vi "live view D01.vi"() -> ()   [LabVIEW 2019, in "D01.lvlib"]
uses:
  D01.lvlib
  <vilib>/userDefined/High Color/IMAQdx.ctl
  <vilib>/vision/Image Controls.llb/IMAQ Image.ctl
  <vilib>/measure/mamon.llb/Trigger Detection for 1 Channel.vi
  <vilib>/measure/NI_MAPro.lvlib
  Calibration Lib.lvlib
  database.lvlib
  <vilib>/vision/driver/NI_Vision_Acquisition_Software.lvlib
panel:
  in  "Verify Calibration1 D01":bool caption="capture grab"
  in  "snapshot":bool
  out "error prj26":errorcluster
  in  "Path":path
  in  "Verify Calibration D01":bool caption="capture grab"
  in  "Close":bool
  in  "Method 2 save D01":bool caption="capture grab"
  in  "Method 1 Save D01":bool caption="Saving txt"
  out "Average Result":string="Average Result"
  out ">18  A":dbl(slide)=1.0 caption=">18 mm" scale=0.0..100.0
  out "16-18  A":dbl(slide)=1.0 caption="16-18 mm" scale=0.0..100.0
  out "14-16  A":dbl(slide)=1.0 caption="14-16 mm" scale=0.0..100.0
  out "12.5-14 A":dbl(slide)=1.0 caption="12.5-14 mm" scale=0.0..100.0
  out "10-12.5  A":dbl(slide)=1.0 caption="10-12.5 mm" scale=0.0..100.0 scale format="%#_4f"
  out "8-10  A":dbl(slide)=1.0 caption="8-10 mm" scale=0.0..100.0
  out "6.3-8  A":dbl(slide)=1.0 caption="6.3-8 mm" scale=0.0..100.0
  out "<6.3  A":dbl(slide)=1.0 caption="<6.3 mm" scale=0.0..100.0
  out "Live Result":string="Live Result"
  out ">18  L":dbl(slide)=1.0 caption=">18 mm" scale=0.0..100.0
  out "Live View":T1(plugin-control) caption="Disc 26"
  out "16-18  L":dbl(slide)=1.0 caption="16-18 mm" scale=0.0..100.0
  out "14-16  L":dbl(slide)=1.0 caption="14-16 mm" scale=0.0..100.0
  out "12.5-14 L":dbl(slide)=1.0 caption="12.5-14 mm" scale=0.0..100.0
  out "10-12.5  L":dbl(slide)=1.0 caption="10-12.5 mm" scale=0.0..100.0 scale format="%#_4f"
  out "8-10  L":dbl(slide)=1.0 caption="8-10 mm" scale=0.0..100.0
  out "6.3-8  L":dbl(slide)=1.0 caption="6.3-8 mm" scale=0.0..100.0
  out "<6.3  L":dbl(slide)=1.0 caption="<6.3 mm" scale=0.0..100.0
  out "disc name":string="Live Info Disc 01"
  out "dsgs":string="DSGS"
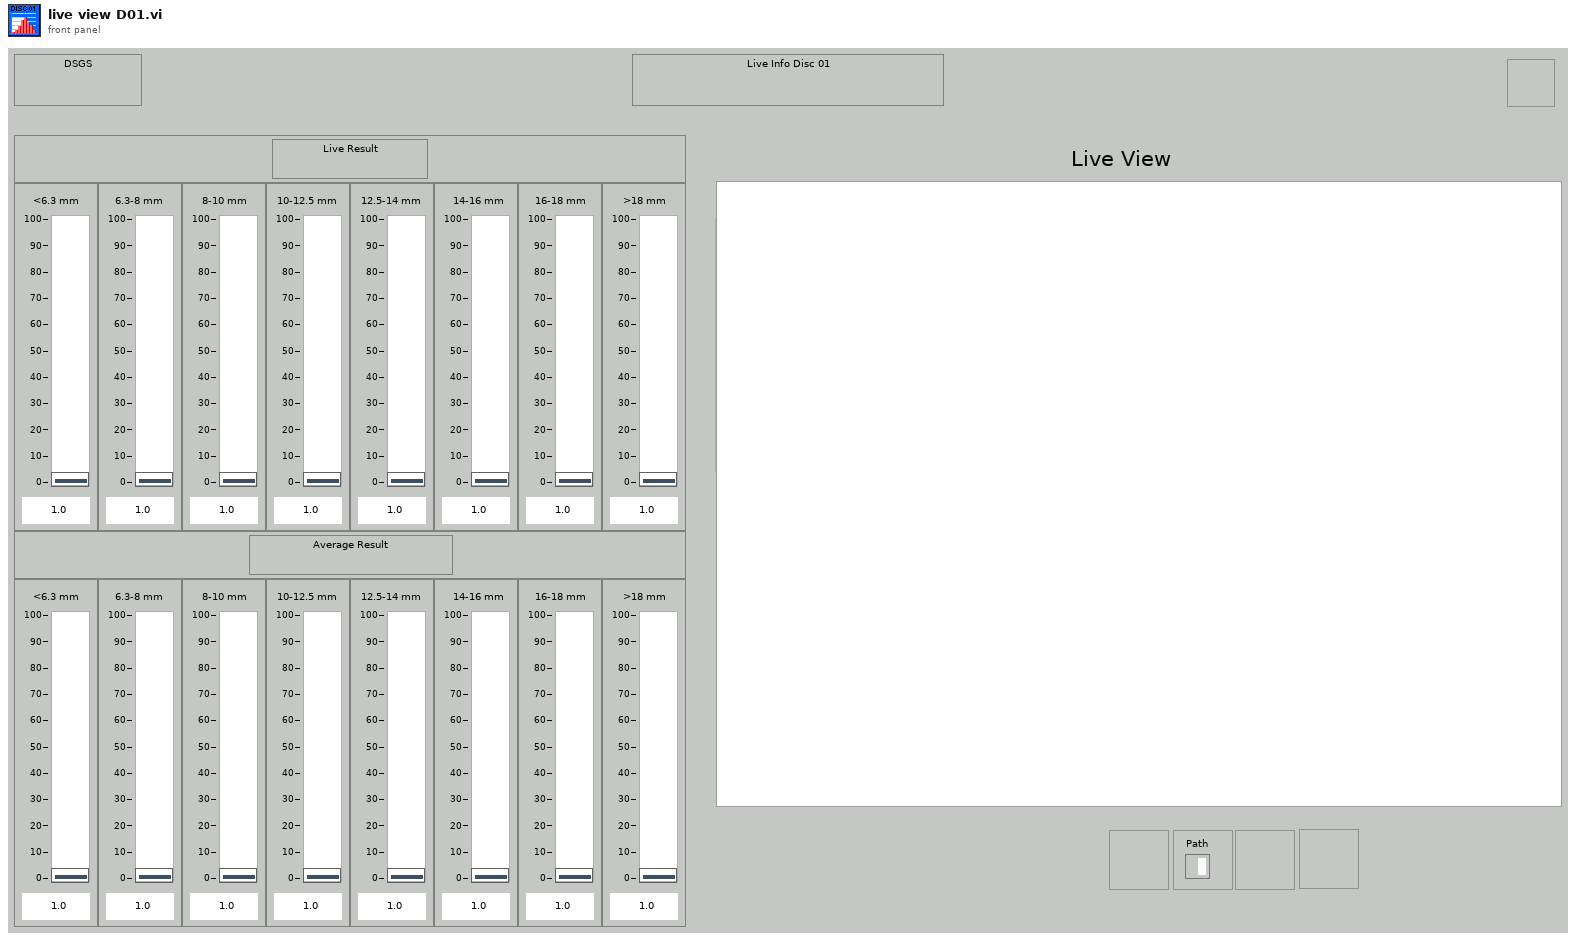
[diagram p1: front panel]
types:
  T1 = typedef "IMAQ Image.ctl" = refnum<image>
  T2 = typedef "IMAQdx.ctl" = refnum<k21>
  T3 = enum8{"Enabled", "Disabled", "Disabled and Grayed Out"}
  T4 = cluster{"date/time string":string, "date/time string":string, "date/time string":string, string, "spreadsheet string":string, string}
  T5 = cluster{"date/time string":string, "date/time string":string, string, "Value":dbl, "Value":dbl, "Value":dbl, "Value":dbl, "Value":dbl, "Value":dbl, "Value":dbl, "Value":dbl}
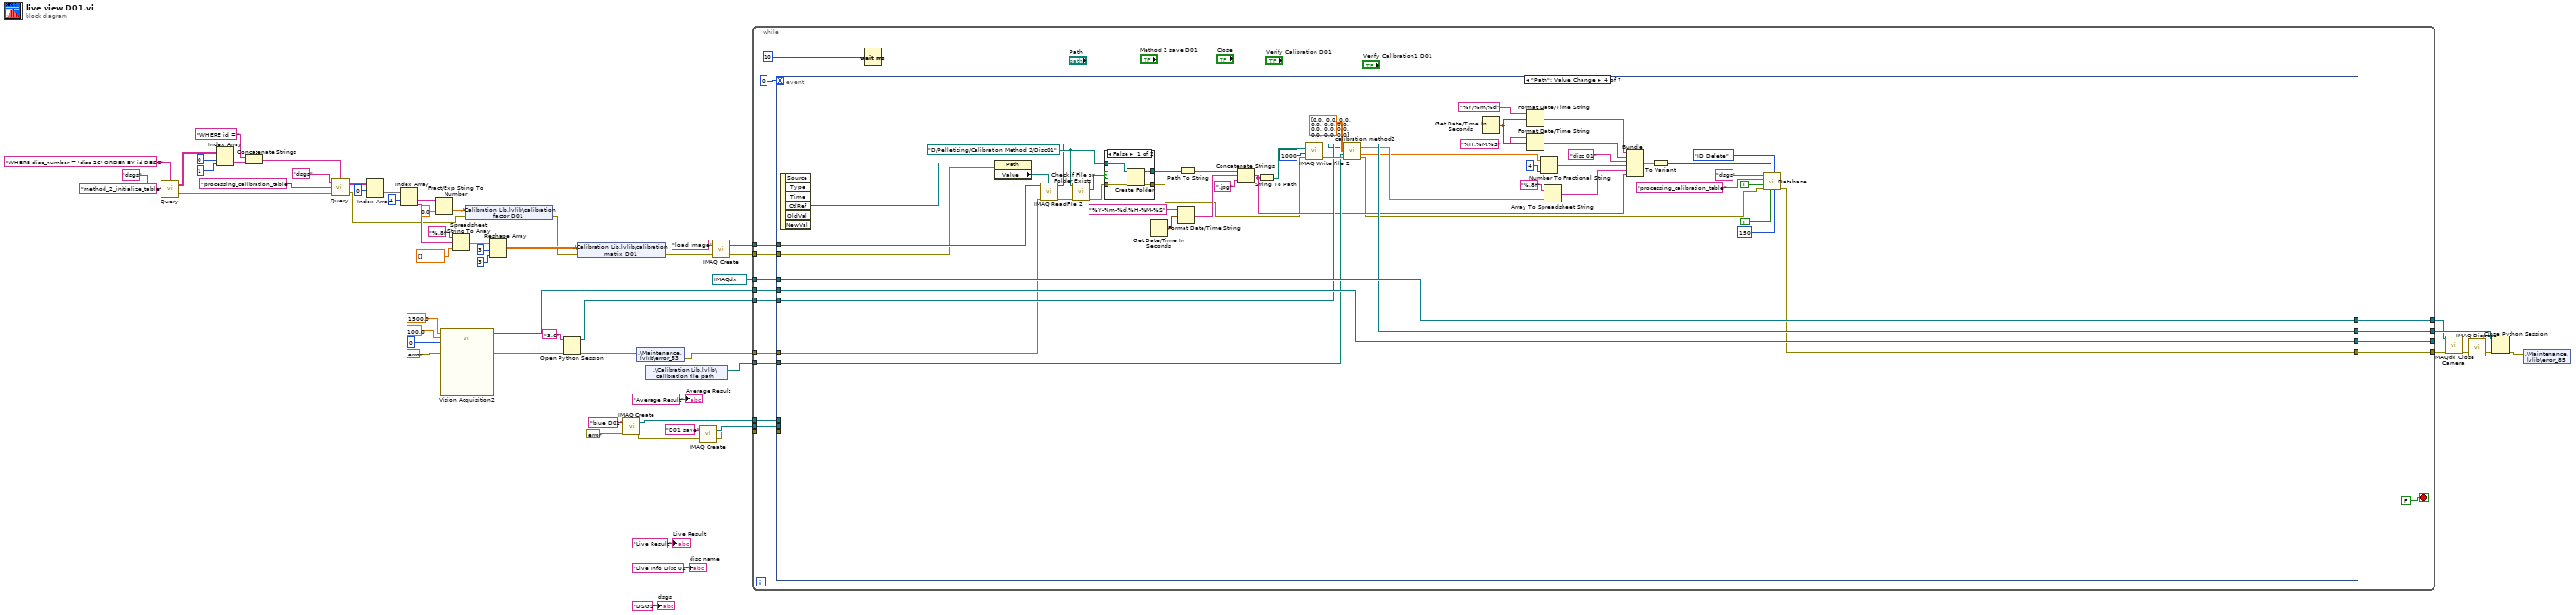
[diagram p0: block diagram]
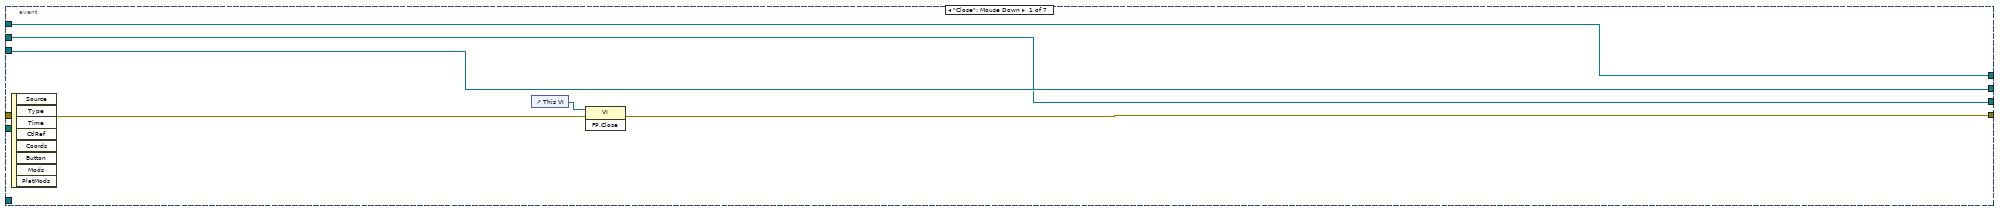
[diagram p2: hidden frame]
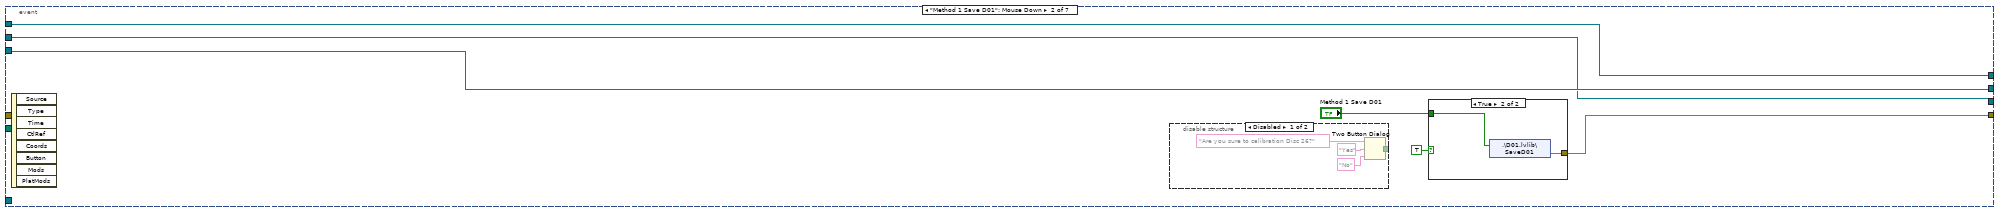
[diagram p3: hidden frame]
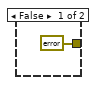
[diagram p5: hidden frame]
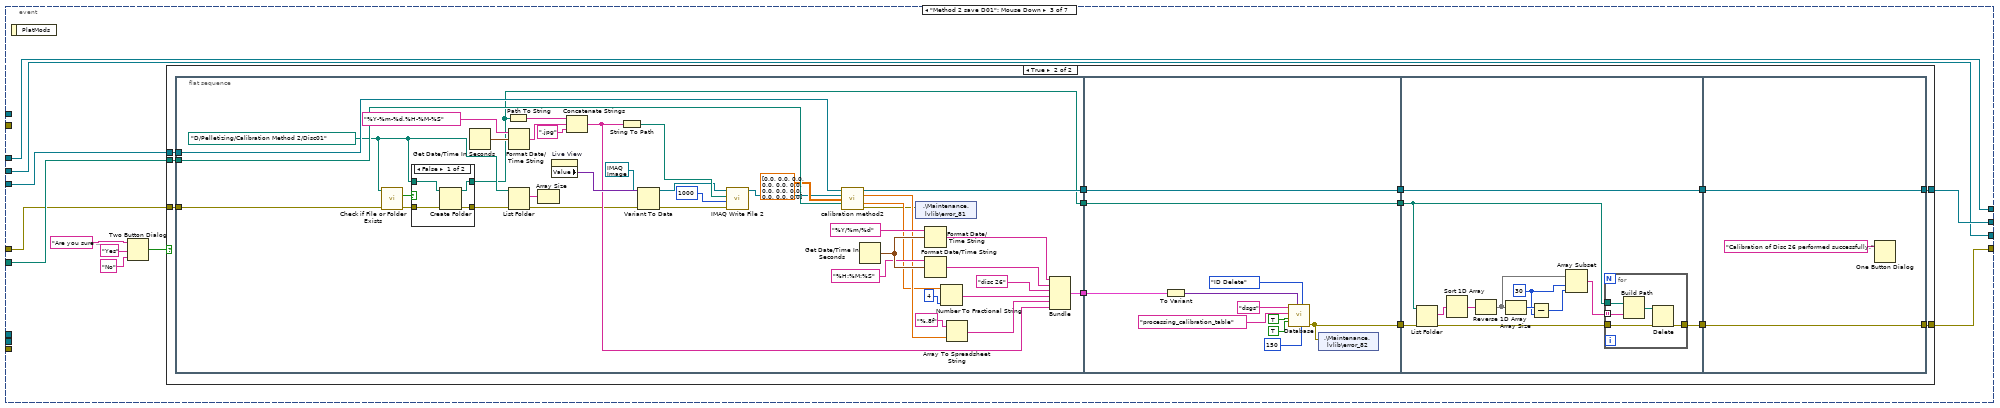
[diagram p6: hidden frame]
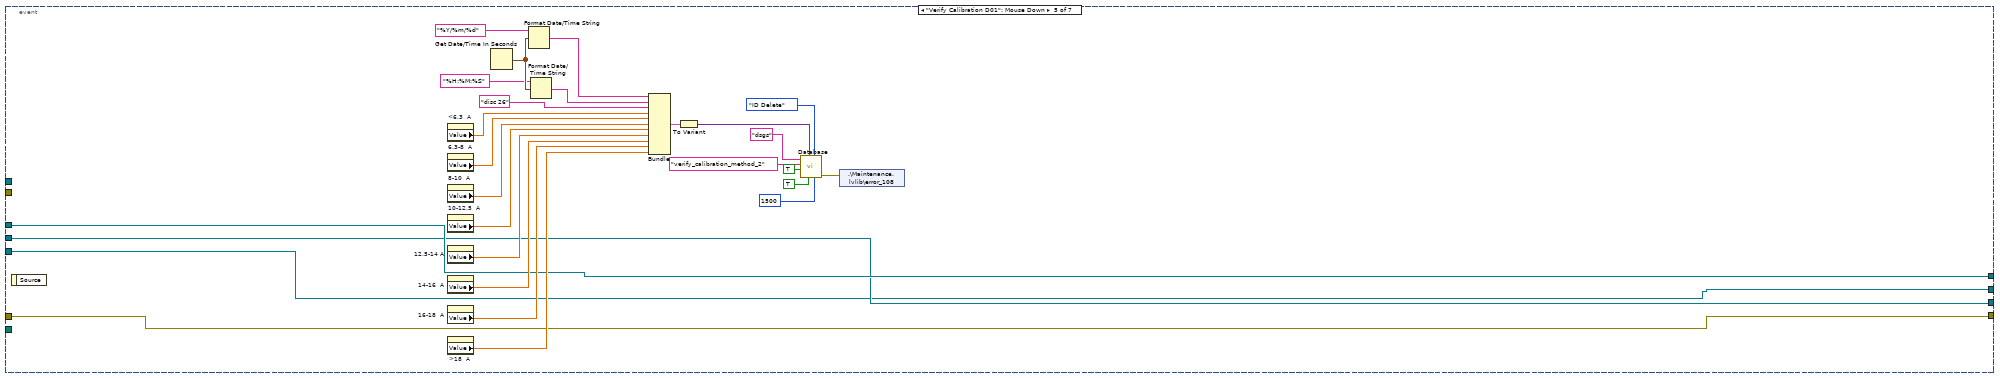
[diagram p10: hidden frame]
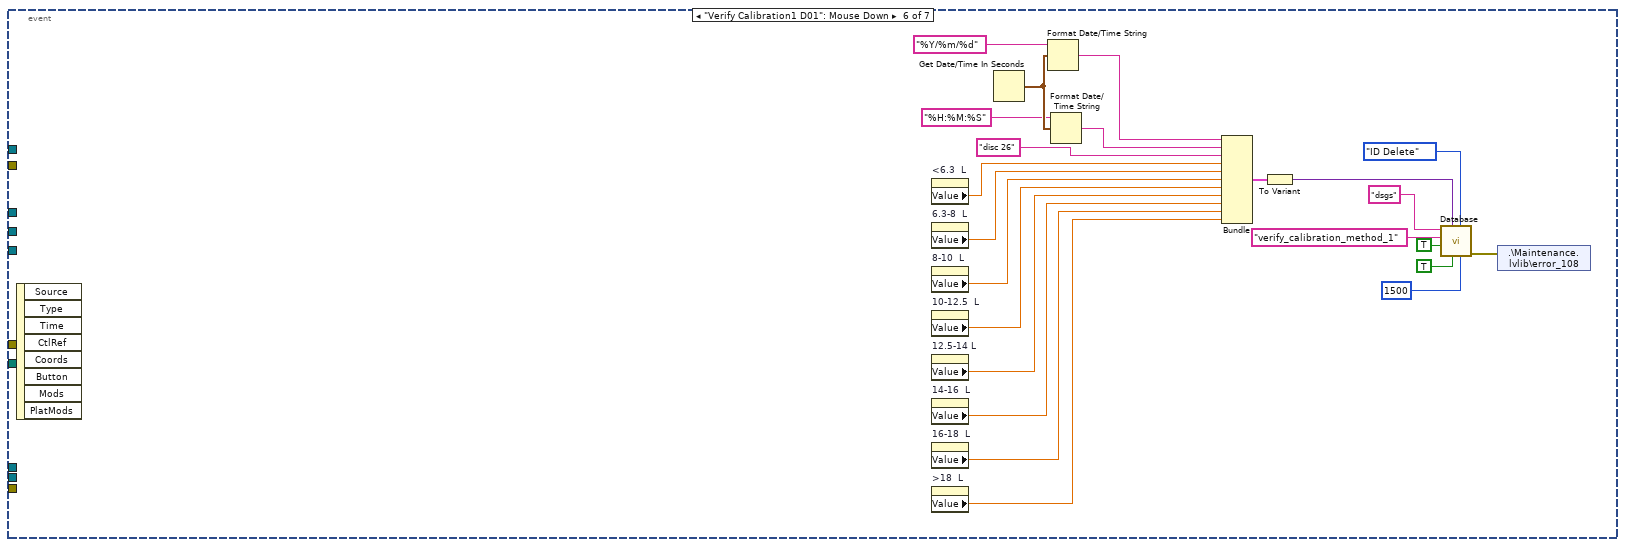
[diagram p11: hidden frame]
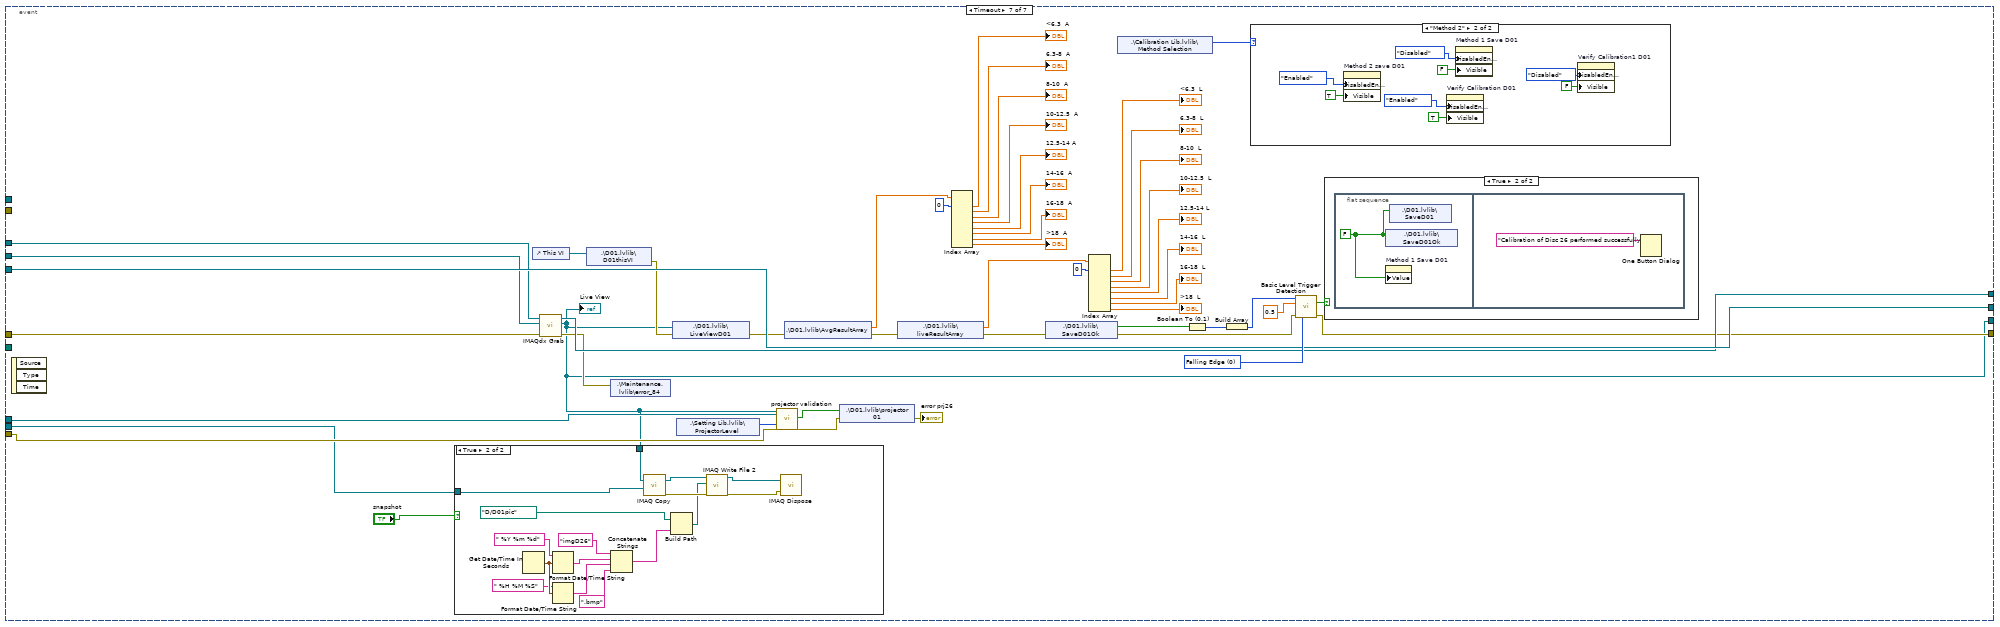
[diagram p12: hidden frame]
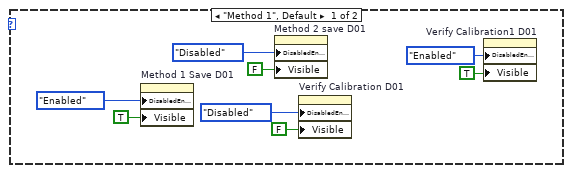
[diagram p14: hidden frame]
diagram:
  n1 = call "Query.vi"("Condition"="WHERE disc_number = 'disc 26' ORDER BY id DESC", "Table Name"="method_2_initialize_table", "Connection Name"="dsgs") -> ("Error out"=w29:errorcluster, "data"=w34:string[][])  [unwired: 1 in]
  n2 = Index Array(array=w34, index (row)=0, index (col)=1 ("disabled index (col)")) -> (element=w27:string)
  n3 = Concatenate Strings("WHERE id = " ("string"), w27) -> (w26:string)
  n4 = call "Query.vi"("Condition"=w26, "Error in"=w29, "Table Name"="processing_calibration_table", "Connection Name"="dsgs") -> ("Error out"=w10:errorcluster, "data"=w25:string[][])
  n5 = Index Array(array=w25, index (row)=0) -> (element=w23:string[])  [unwired: 1 in]
  n6 = Index Array(array=w23, index #1=4 ("index")) -> (element #1=w21:string, element #2=w13:string)  [unwired: 1 in]
  n7 = Fract/Exp String To Number(string=w21, default (0 dbl)=sgl 0.0 ("default (0 DBL)")) -> (number=w20:sgl)  [unwired: 2 in, 1 out]
  n8 = call "Vision Acquisition2"("Exposure Time (Abs)"=1500.0, "Acquisition Frame Rate (Abs)"=100.0, "Gain (Raw) Upper Limit"=i64 0, "error in"=errorcluster {"status"=FALSE, "code"=0, "source"=""}) -> ("Image Out"=w49:T1, "error out"=w8:errorcluster)  [unwired: 21 in, 1 out]
  n9 = Spreadsheet String To Array(format string="%.8f", spreadsheet string=w13, array type (2D Dbl)=sgl[] []) -> (array=w17:sgl[])  [unwired: 1 in]
  n10 = shared-variable ".\\Calibration Lib.lvlib\\calibration factor D01"(w20, error in=w10) -> (error out=w11:errorcluster)
  n11 = Reshape Array(w17, 3 ("dimension size"), 3 ("dimension size")) -> (w12:sgl[][])
  n12 = Open Python Session(python version="3.6" ("Python version"), 3:w8) -> (session out=w56:refnum<k35>, error out=w43:errorcluster)  [unwired: 1 in]
  n13 = shared-variable ".\\Calibration Lib.lvlib\\calibration matrix D01"(w12, error in=w11) -> (error out=w9:errorcluster)
  n14 = call "IMAQ Create"("Image Name"="blue D01", "error in (no error)"=errorcluster {"status"=FALSE, "code"=0, "source"=""}) -> ("New Image"=w6:T1, "error out"=w4:errorcluster)  [unwired: 3 in]
  n15 = shared-variable ".\\Maintenance.lvlib\\error_83"(w43) -> (error out=w41:errorcluster)  [unwired: 1 in]
  n16 = shared-variable ".\\Calibration Lib.lvlib\\calibration file path"() -> (w44:path)  [unwired: 1 in, 1 out]
  n17 = call "IMAQ Create"("Image Name"="D01 save", "error in (no error)"=w4) -> ("New Image"=w1:T1, "error out"=w3:errorcluster)  [unwired: 3 in]
  n18 = call "IMAQ Create"("Image Name"="load image", "error in (no error)"=w9) -> ("New Image"=w38:T1, "error out"=w39:errorcluster)  [unwired: 3 in]
  n19 = while {
    tunnel: w56 -> [w76]
    tunnel: w44 -> [w75]
    tunnel: w41 -> [w74]
    tunnel: w49 -> [w72]
    tunnel: [w71] -> w53
    tunnel: [w70] -> w55
    tunnel: [w69] -> _
    tunnel: T2 "disc01" ("Session In") -> [w68]
    tunnel: [w67] -> w50
    tunnel: w39 -> [w66]
    tunnel: w38 -> [w65]
    tunnel: w6 -> [w64]
    tunnel: w3 -> [w63]
    tunnel: w1 -> [w62]
    stop <- FALSE stop-if-true
    n20 = event shown="[3] \"Path\": Value Change" {
      selector: _ -> [_ _ _ _ _ _ _]
      dyn-events: _ -> [_ _ _ _ _ _ _]
      timeout: 0 -> [_ _ _ _ _ _ _]
      tunnel: w76 -> [w81 w89 w107 w234 w258 _ w325]
      tunnel: w75 -> [_ _ w108 w233 _ _ _]
      tunnel: [w83 w90 w102 w202 w261 _ w319] -> w71
      tunnel: w74 -> [w82 _ w106 w228 w261 _ w323]
      tunnel: w72 -> [w80 w88 w104 w248 w259 _ w309]
      tunnel: [w81 w89 w105 w232 w258 _ w325] -> w70
      tunnel: [w80 w88 w104 w248 w259 _ w306] -> w69
      tunnel: w68 -> [w79 w87 w103 w249 w260 _ w310]
      tunnel: [w79 w87 w103 w249 w260 _ w322] -> w67
      tunnel: w66 -> [_ _ _ w227 _ _ _]
      tunnel: w65 -> [_ _ _ w229 _ _ _]
      tunnel: w64 -> [_ _ _ _ _ _ w316]
      tunnel: w63 -> [_ _ _ _ _ _ w312]
      tunnel: w62 -> [_ _ _ _ _ _ w307]
      event "Close": Mouse Down {
        n21 = event-data() -> ()  [unwired: 1 in, 8 out]
        n22 = control-ref of="This VI"() -> (w84:refnum<vi>)
        n23 = invoke class="VI" method="FP.Close"(reference=w84, error in=w82) -> (error out=w83:errorcluster)  [unwired: 1 in, 2 out]
      }
      event "Method 1 Save D01": Mouse Down {
        n24 = event-data() -> ()  [unwired: 1 in, 8 out]
        n25 = disable-structure shown="Disabled" {
          disable-tunnel: [w91 _] -> _
          frame Disabled {
            n26 = Two Button Dialog(message="Are you sure to calibration Disc 26?", 1:"No" ("F button name (\"Cancel\")"), 2:"Yes" ("T button name (\"OK\")")) -> (T button?=w91:bool)
          }
          frame Enabled {
          }
        }
        n27 = case shown="True" TRUE {
          tunnel: [errorcluster {"status"=FALSE, "code"=0, "source"=""} ("error IO") w97] -> w90
          tunnel: "Method 1 Save D01" -> [_ w96]
          frame False {
          }
          frame True {
            n28 = shared-variable ".\\D01.lvlib\\SaveD01"(w96) -> (error out=w97:errorcluster)  [unwired: 1 in]
          }
        }
      }
      event "Method 2 save D01": Mouse Down {
        n29 = event-data() -> ()  [unwired: 1 in, 1 out]
        n30 = Two Button Dialog(message="Are you sure to calibration Disc 26?", 1:"No" ("F button name (\"Cancel\")"), 2:"Yes" ("T button name (\"OK\")")) -> (T button?=w98:bool)
        n31 = case shown="True" w98 {
          tunnel: w108 -> [_ w117]
          tunnel: w107 -> [w109 w116]
          tunnel: w106 -> [w110 w115]
          tunnel: [w109 w114] -> w105
          tunnel: [w110 w113] -> w102
          frame False {
          }
          frame True {
            n32 = flat-sequence {
              tunnel: [w162] -> w123
              tunnel: [w153] -> w122
              tunnel: w115 -> [w135]
              tunnel: w116 -> [w151]
              tunnel: w117 -> [w152]
              tunnel: [w126] -> w121
              tunnel: w123 -> [w179]
              tunnel: w122 -> [w174]
              tunnel: [w179] -> w120
              tunnel: w121 -> [w170]
              tunnel: [w170] -> w119
              tunnel: [w169] -> w118
              tunnel: w120 -> [w191]
              tunnel: w119 -> [w183]
              tunnel: w118 -> [w182]
              tunnel: [w191] -> w112
              tunnel: [w181] -> w111
              tunnel: [w198] -> w113
              tunnel: [w199] -> w114
              tunnel: w112 -> [w199]
              tunnel: w111 -> [w198]
              frame #0 {
                w127 = path "D:/Pelletizing/Calibration Method 2/Disc01" ("path")
                n33 = call <vilib>:"Check if File or Folder Exists.vi"("error in (no error)"=w135, "path"=w127) -> ("error out"=w136:errorcluster, "file or folder exists?"=w137:bool)  [unwired: 7 in, 1 out]
                n34 = case shown="False" w137 {
                  tunnel: [w164 w168] -> w126
                  tunnel: w127 -> [w166 w168]
                  tunnel: w136 -> [w165 w167]
                  tunnel: [w163 w167] -> w129
                  frame False {
                    n35 = Create Folder(path (use dialog)=w166, error in=w165) -> (created path=w164:path, error out=w163:errorcluster)  [unwired: 1 in, 1 out]
                  }
                  frame True {
                  }
                }
                n36 = Get Date/Time In Seconds() -> (seconds since 1Jan1904=w141:timestamp)
                n37 = Path To String(path=w126) -> (string=w131:string)
                n38 = Format Date/Time String(time format string (%c)="%Y-%m-%d,%H-%M-%S", seconds (now)=w141) -> (date/time string=w139:string)  [unwired: 1 in]
                n39 = List Folder(path=w127, error in=w129) -> (filenames=w130:string[], error out=w128:errorcluster)  [unwired: 2 in, 2 out]
                n40 = Array Size(array=w130) -> ()  [unwired: 1 out]
                n41 = property on="Live View" class="ImageControl"() -> ("Value"=w150:variant)  [unwired: 2 in, 2 out]
                n42 = Concatenate Strings(w131, w139, ".jpg" ("string")) -> (w133:string)
                n43 = String To Path(string=w133) -> (path=w134:path)
                n44 = Variant To Data(error in=w128, type=T1 refnum ("New Image"), Variant=w150) -> (data=w124:T1, error out=w142:errorcluster)
                n45 = call-poly "IMAQ Write File 2"("error in (no error)"=w142, "Image Quality"=u32 1000, "File Path"=w134, "Image"=w124) -> ("Image Out (duplicate)"=w125:T1)  [unwired: 6 in, 1 out]
                n46 = call "calibration method2.vi"("session in"=w151, "Image IN"=w125, "initialize matrix"=sgl[][] [[0.0, 0.0, 0.0], [0.0, 0.0, 0.0], [0.0, 0.0, 0.0], [0.0, 0.0, 0.0]] ("(4*3) array"), "module path"=w152) -> ("session out"=w162:refnum<k35>, "calibration vector"=w146:sgl[], "factor"=w144:sgl, "error out"=w132:errorcluster)  [unwired: 7 in, 1 out]
                n47 = Get Date/Time In Seconds() -> (seconds since 1Jan1904=w159:timestamp)
                n48 = shared-variable ".\\Maintenance.lvlib\\error_81"(w132) -> ()  [unwired: 1 in, 1 out]
                n49 = Format Date/Time String(time format string (%c)="%Y/%m/%d", seconds (now)=w159) -> (date/time string=w160:string)  [unwired: 1 in]
                n50 = Format Date/Time String(time format string (%c)="%H:%M:%S", seconds (now)=w159) -> (date/time string=w161:string)  [unwired: 1 in]
                n51 = Number To Fractional String(number=w144, precision (6)=i16 4) -> (F-format string=w155:string)  [unwired: 2 in]
                n52 = Array To Spreadsheet String(array=w146, 3:"%.8f" ("format string")) -> (spreadsheet string=w154:string)  [unwired: 1 in]
                n53 = Bundle("date/time string"=w160, "date/time string"=w161, "date/time string"="disc 26", w155, "spreadsheet string"=w154, w133) -> (w153:T4)  [unwired: 1 in]
              }
              frame #1 {
                n54 = To Variant(anything=w174) -> (Variant=w173:variant)
                n55 = call "Database.vi"("Maximum Row"=150, "Enum"=enum16{"ID Delete", "Time Delete"}."ID Delete", "Delete row?"=TRUE, "Data"=w173, "Auto Increment ID?"=TRUE, "Table"="processing_calibration_table", "Connection"="dsgs") -> ("Error out"=w169:errorcluster)  [unwired: 4 in]
                n56 = shared-variable ".\\Maintenance.lvlib\\error_82"(w169) -> ()  [unwired: 1 in, 1 out]
              }
              frame #2 {
                w184 = 30 ("index")
                n57 = List Folder(path=w183, error in=w182) -> (filenames=w190:string[], error out=w180:errorcluster)  [unwired: 2 in, 2 out]
                n58 = Sort 1D Array(array=w190) -> (sorted array=w189:string[])
                n59 = Reverse 1D Array(array=w189) -> (reversed array=w188:string[])
                n60 = Array Size(array=w188) -> (size(s)=w187:i32)
                n61 = Subtract(x=w187, y=w184) -> (x-y=w186:i32)
                n62 = Array Subset(array=w188, index=w184, length=w186) -> (w185:string[])
                n63 = for {
                  tunnel: w185 -> [w195] mode=indexing
                  tunnel: w183 -> [w196]
                  tunnel: [w193] -> w181
                  tunnel: w180 -> [w192]
                  n64 = Build Path(base path=w196, name or relative path=w195) -> (appended path=w194:path)
                  n65 = Delete(path (use dialog)=w194, error in=w192) -> (error out=w193:errorcluster)  [unwired: 3 in, 2 out]
                }
              }
              frame #3 {
                n66 = One Button Dialog(message="Calibration of Disc 26 performed successfully.") -> ()  [unwired: 1 in, 1 out]
              }
            }
          }
        }
      }
      event "Path": Value Change {
        w239 = path "D:/Pelletizing/Calibration Method 2/Disc01" ("path")
        n67 = event-data() -> ("CtlRef"=w231:refnum<vi>)  [unwired: 1 in, 5 out]
        n68 = property class="Path"(reference=w231, error in=w227) -> ("Value"=w230:path)  [unwired: 2 out]
        n69 = call "IMAQ ReadFile 2"("File Path"=w230, "error in (no error)"=w228, "Image"=w229) -> ("error out"=w225:errorcluster, "Image Out"=w226:T1)  [unwired: 4 in, 3 out]
        n70 = call <vilib>:"Check if File or Folder Exists.vi"("error in (no error)"=w225, "path"=w239) -> ("error out"=w236:errorcluster, "file or folder exists?"=w240:bool)  [unwired: 7 in, 1 out]
        n71 = case shown="False" w240 {
          tunnel: [w251 w255] -> w238
          tunnel: w239 -> [w253 w255]
          tunnel: w236 -> [w252 w254]
          tunnel: [w250 w254] -> w201
          frame False {
            n72 = Create Folder(path (use dialog)=w253, error in=w252) -> (created path=w251:path, error out=w250:errorcluster)  [unwired: 1 in, 1 out]
          }
          frame True {
          }
        }
        n73 = Get Date/Time In Seconds() -> (seconds since 1Jan1904=w244:timestamp)
        n74 = Format Date/Time String(time format string (%c)="%Y-%m-%d,%H-%M-%S", seconds (now)=w244) -> (date/time string=w242:string)  [unwired: 1 in]
        n75 = Path To String(path=w238) -> (string=w237:string)
        n76 = Concatenate Strings(w237, w242, ".jpg" ("string")) -> (w213:string)
        n77 = String To Path(string=w213) -> (path=w235:path)
        n78 = call-poly "IMAQ Write File 2"("error in (no error)"=w201, "Image Quality"=u32 1000, "File Path"=w235, "Image"=w226) -> ("error out"=w246:errorcluster, "Image Out (duplicate)"=w224:T1)  [unwired: 6 in]
        n79 = call "calibration method2.vi"("session in"=w234, "Image IN"=w224, "initialize matrix"=sgl[][] [[0.0, 0.0, 0.0], [0.0, 0.0, 0.0], [0.0, 0.0, 0.0], [0.0, 0.0, 0.0]] ("(4*3) array"), "module path"=w233, "error in"=w246) -> ("session out"=w232:refnum<k35>, "calibration vector"=w212:sgl[], "factor"=w211:sgl, "error out"=w200:errorcluster)  [unwired: 6 in, 1 out]
        n80 = Get Date/Time In Seconds() -> (seconds since 1Jan1904=w221:timestamp)
        n81 = Format Date/Time String(time format string (%c)="%Y/%m/%d", seconds (now)=w221) -> (date/time string=w222:string)  [unwired: 1 in]
        n82 = Format Date/Time String(time format string (%c)="%H:%M:%S", seconds (now)=w221) -> (date/time string=w223:string)  [unwired: 1 in]
        n83 = Number To Fractional String(number=w211, precision (6)=i16 4) -> (F-format string=w217:string)  [unwired: 2 in]
        n84 = Array To Spreadsheet String(array=w212, 3:"%.8f" ("format string")) -> (spreadsheet string=w216:string)  [unwired: 1 in]
        n85 = Bundle("date/time string"=w222, "date/time string"=w223, "date/time string"="disc 01", w217, "spreadsheet string"=w216, w213) -> (w203:T4)  [unwired: 1 in]
        n86 = To Variant(anything=w203) -> (Variant=w206:variant)
        n87 = call "Database.vi"("Maximum Row"=150, "Enum"=enum16{"ID Delete", "Time Delete"}."ID Delete", "Delete row?"=TRUE, "Data"=w206, "Error in"=w200, "Auto Increment ID?"=TRUE, "Table"="processing_calibration_table", "Connection"="dsgs") -> ("Error out"=w202:errorcluster)  [unwired: 3 in]
      }
      event "Verify Calibration D01": Mouse Down {
        n88 = event-data() -> ()  [unwired: 1 in, 1 out]
        n89 = property on="<6.3  A" class="Slide (strict)"() -> ("Value"=w276:dbl)  [unwired: 2 in, 2 out]
        n90 = property on="6.3-8  A" class="Slide (strict)"() -> ("Value"=w275:dbl)  [unwired: 2 in, 2 out]
        n91 = property on="8-10  A" class="Slide (strict)"() -> ("Value"=w274:dbl)  [unwired: 2 in, 2 out]
        n92 = property on="10-12.5  A" class="Slide (strict)"() -> ("Value"=w273:dbl)  [unwired: 2 in, 2 out]
        n93 = property on="12.5-14 A" class="Slide (strict)"() -> ("Value"=w272:dbl)  [unwired: 2 in, 2 out]
        n94 = property on="14-16  A" class="Slide (strict)"() -> ("Value"=w271:dbl)  [unwired: 2 in, 2 out]
        n95 = property on="16-18  A" class="Slide (strict)"() -> ("Value"=w270:dbl)  [unwired: 2 in, 2 out]
        n96 = property on=">18  A" class="Slide (strict)"() -> ("Value"=w269:dbl)  [unwired: 2 in, 2 out]
        n97 = Get Date/Time In Seconds() -> (seconds since 1Jan1904=w281:timestamp)
        n98 = Format Date/Time String(time format string (%c)="%Y/%m/%d", seconds (now)=w281) -> (date/time string=w279:string)  [unwired: 1 in]
        n99 = Format Date/Time String(time format string (%c)="%H:%M:%S", seconds (now)=w281) -> (date/time string=w278:string)  [unwired: 1 in]
        n100 = Bundle("date/time string"=w279, "date/time string"=w278, "disc 26", "Value"=w276, "Value"=w275, "Value"=w274, "Value"=w273, "Value"=w272, "Value"=w271, "Value"=w270, "Value"=w269) -> (w268:T5)  [unwired: 1 in]
        n101 = To Variant(anything=w268) -> (Variant=w267:variant)
        n102 = call "Database.vi"("Maximum Row"=1500, "Enum"=enum16{"ID Delete", "Time Delete"}."ID Delete", "Delete row?"=TRUE, "Data"=w267, "Auto Increment ID?"=TRUE, "Table"="verify_calibration_method_2", "Connection"="dsgs") -> ("Error out"=w262:errorcluster)  [unwired: 4 in]
        n103 = shared-variable ".\\Maintenance.lvlib\\error_108"(w262) -> ()  [unwired: 1 in, 1 out]
      }
      event "Verify Calibration1 D01": Mouse Down {
        n104 = event-data() -> ()  [unwired: 1 in, 8 out]
        n105 = property on="<6.3  L" class="Slide (strict)"() -> ("Value"=w299:dbl)  [unwired: 2 in, 2 out]
        n106 = property on="6.3-8  L" class="Slide (strict)"() -> ("Value"=w298:dbl)  [unwired: 2 in, 2 out]
        n107 = property on="8-10  L" class="Slide (strict)"() -> ("Value"=w297:dbl)  [unwired: 2 in, 2 out]
        n108 = property on="10-12.5  L" class="Slide (strict)"() -> ("Value"=w296:dbl)  [unwired: 2 in, 2 out]
        n109 = property on="12.5-14 L" class="Slide (strict)"() -> ("Value"=w295:dbl)  [unwired: 2 in, 2 out]
        n110 = property on="14-16  L" class="Slide (strict)"() -> ("Value"=w294:dbl)  [unwired: 2 in, 2 out]
        n111 = property on="16-18  L" class="Slide (strict)"() -> ("Value"=w293:dbl)  [unwired: 2 in, 2 out]
        n112 = property on=">18  L" class="Slide (strict)"() -> ("Value"=w292:dbl)  [unwired: 2 in, 2 out]
        n113 = Get Date/Time In Seconds() -> (seconds since 1Jan1904=w304:timestamp)
        n114 = Format Date/Time String(time format string (%c)="%Y/%m/%d", seconds (now)=w304) -> (date/time string=w302:string)  [unwired: 1 in]
        n115 = Format Date/Time String(time format string (%c)="%H:%M:%S", seconds (now)=w304) -> (date/time string=w301:string)  [unwired: 1 in]
        n116 = Bundle("date/time string"=w302, "date/time string"=w301, "disc 26", "Value"=w299, "Value"=w298, "Value"=w297, "Value"=w296, "Value"=w295, "Value"=w294, "Value"=w293, "Value"=w292) -> (w291:T5)  [unwired: 1 in]
        n117 = To Variant(anything=w291) -> (Variant=w290:variant)
        n118 = call "Database.vi"("Maximum Row"=1500, "Enum"=enum16{"ID Delete", "Time Delete"}."ID Delete", "Delete row?"=TRUE, "Data"=w290, "Auto Increment ID?"=TRUE, "Table"="verify_calibration_method_1", "Connection"="dsgs") -> ("Error out"=w285:errorcluster)  [unwired: 4 in]
        n119 = shared-variable ".\\Maintenance.lvlib\\error_108"(w285) -> ()  [unwired: 1 in, 1 out]
      }
      event Timeout {
        w330 = u16 0 items=["Falling Edge", "Rising Edge"] ("trigger slope")
        n120 = event-data() -> ()  [unwired: 1 in, 3 out]
        n121 = control-ref of="This VI"() -> (w324:refnum<vi>)
        n122 = call <vilib>:"IMAQdx Grab.vi"("error in"=w323, "Image In"=w309, "Session In"=w310) -> ("error out"=w318:errorcluster, "Image Out"=w306:T1, "Session Out"=w322:T2)  [unwired: 1 in, 5 out]
        "Live View" <- w306
        n123 = case shown="True" "snapshot" {
          tunnel: w307 -> [_ w370]
          tunnel: w306 -> [_ w369]
          frame False {
          }
          frame True {
            n124 = Get Date/Time In Seconds() -> (seconds since 1Jan1904=w363:timestamp)
            n125 = Format Date/Time String(time format string (%c)=" %Y %m %d", seconds (now)=w363) -> (date/time string=w359:string)  [unwired: 1 in]
            n126 = Format Date/Time String(time format string (%c)=" %H %M %S", seconds (now)=w363) -> (date/time string=w358:string)  [unwired: 1 in]
            n127 = Concatenate Strings("imgD26" ("string"), w359, w358, ".bmp" ("string")) -> (w356:string)
            n128 = call "IMAQ Copy"("Image Dst"=w370, "Image Src"=w369) -> ("error out"=w367:errorcluster, "Image Dst Out"=w368:T1)  [unwired: 4 in]
            n129 = Build Path(base path=path "D:/D01pic" ("File Path"), name or relative path=w356) -> (appended path=w355:path)
            n130 = call-poly "IMAQ Write File 2"("error in (no error)"=w367, "File Path"=w355, "Image"=w368) -> ("error out"=w365:errorcluster, "Image Out (duplicate)"=w366:T1)  [unwired: 7 in]
            n131 = call "IMAQ Dispose"("Image"=w366, "error in (no error)"=w365) -> ()  [unwired: 4 in, 1 out]
          }
        }
        n132 = shared-variable ".\\D01.lvlib\\D01thisVI"(w324) -> (error out=w317:errorcluster)  [unwired: 1 in]
        n133 = shared-variable ".\\Maintenance.lvlib\\error_84"(w318) -> ()  [unwired: 1 in, 1 out]
        n134 = shared-variable ".\\D01.lvlib\\LiveViewD01"(w306, error in=w317) -> (error out=w321:errorcluster)
        n135 = shared-variable ".\\Setting Lib.lvlib\\ProjectorLevel"() -> (w311:i32)  [unwired: 1 in, 1 out]
        n136 = call "projector validation.vi"("Image Src"=w306, "blue channel"=w316, "on/off level"=w311, "error in (no error)"=w312) -> ("on/off"=w315:bool, "error out"=w314:errorcluster)  [unwired: 14 in]
        n137 = shared-variable ".\\D01.lvlib\\AvgResultArray"(error in=w321) -> (w345:dbl[], error out=w327:errorcluster)
        n138 = shared-variable ".\\D01.lvlib\\projector 01"(w315, error in=w314) -> (error out=→"error prj26":errorcluster)
        n139 = shared-variable ".\\D01.lvlib\\liveResultArray"(error in=w327) -> (w344:dbl[], error out=w326:errorcluster)
        n140 = Index Array(array=w345, index #1=0 ("index")) -> (element #1=→"<6.3  A":dbl, element #2=→"6.3-8  A":dbl, element #3=→"8-10  A":dbl, element #4=→"10-12.5  A":dbl, element #5=→"12.5-14 A":dbl, element #6=→"14-16  A":dbl, element #7=→"16-18  A":dbl, element #8=→">18  A":dbl)  [unwired: 7 in]
        n141 = shared-variable ".\\D01.lvlib\\SaveD01Ok"(error in=w326) -> (w331:bool, error out=w320:errorcluster)
        n142 = Index Array(array=w344, index #1=0 ("index")) -> (element #1=→"<6.3  L":dbl, element #2=→"6.3-8  L":dbl, element #3=→"8-10  L":dbl, element #4=→"10-12.5  L":dbl, element #5=→"12.5-14 L":dbl, element #6=→"14-16  L":dbl, element #7=→"16-18  L":dbl, element #8=→">18  L":dbl)  [unwired: 7 in]
        n143 = shared-variable ".\\Calibration Lib.lvlib\\Method Selection"() -> (w328:enum32{"Method 1", "Method 2"})  [unwired: 1 in, 1 out]
        n144 = Boolean To (0,1)(Boolean=w331) -> (0, 1=w334:i16)
        n145 = Build Array(w334) -> (w333:i16[])
        n146 = case shown="\"Method 2\"" w328 {
          frame "Method 1", Default {
            n147 = property on="Method 1 Save D01" class="Bool (strict)"("DisabledEnum"=T3."Enabled" ("Disabled"), "Visible"=TRUE) -> ()  [unwired: 2 in, 2 out]
            n148 = property on="Method 2 save D01" class="Bool (strict)"("DisabledEnum"=T3."Disabled" ("Disabled"), "Visible"=FALSE) -> ()  [unwired: 2 in, 2 out]
            n149 = property on="Verify Calibration D01" class="Bool (strict)"("DisabledEnum"=T3."Disabled" ("Disabled"), "Visible"=FALSE) -> ()  [unwired: 2 in, 2 out]
            n150 = property on="Verify Calibration1 D01" class="Bool (strict)"("DisabledEnum"=T3."Enabled" ("Disabled"), "Visible"=TRUE) -> ()  [unwired: 2 in, 2 out]
          }
          frame "Method 2" {
            n151 = property on="Method 2 save D01" class="Bool (strict)"("DisabledEnum"=T3."Enabled" ("Disabled"), "Visible"=TRUE) -> ()  [unwired: 2 in, 2 out]
            n152 = property on="Verify Calibration D01" class="Bool (strict)"("DisabledEnum"=T3."Enabled" ("Disabled"), "Visible"=TRUE) -> ()  [unwired: 2 in, 2 out]
            n153 = property on="Method 1 Save D01" class="Bool (strict)"("DisabledEnum"=T3."Disabled" ("Disabled"), "Visible"=FALSE) -> ()  [unwired: 2 in, 2 out]
            n154 = property on="Verify Calibration1 D01" class="Bool (strict)"("DisabledEnum"=T3."Disabled" ("Disabled"), "Visible"=FALSE) -> ()  [unwired: 2 in, 2 out]
          }
        }
        n155 = call-poly <vilib>:"Basic Level Trigger Detection.vi"("signal in"=w333, "level"=0.5, "error in (no error)"=w320, "trigger slope"=w330) -> ("trigger detected?"=w329:bool, "error out"=w319:errorcluster)  [unwired: 9 in, 1 out]
        n156 = case shown="True" w329 {
          frame False {
          }
          frame True {
            n157 = flat-sequence {
              frame #0 {
                w387 = FALSE
                n158 = shared-variable ".\\D01.lvlib\\SaveD01Ok"(w387) -> ()  [unwired: 1 in, 1 out]
                n159 = property on="Method 1 Save D01" class="Bool (strict)"("Value"=w387) -> ()  [unwired: 2 in, 2 out]
                n160 = shared-variable ".\\D01.lvlib\\SaveD01"(w387) -> ()  [unwired: 1 in, 1 out]
              }
              frame #1 {
                n161 = One Button Dialog(message="Calibration of Disc 26 performed successfully.") -> ()  [unwired: 1 in, 1 out]
              }
            }
          }
        }
      }
    }
    n162 = Wait (ms)(milliseconds to wait=u32 10) -> ()  [unwired: 1 out]
  }
  n163 = call <vilib>:"IMAQdx Close Camera.vi"("error in"=w53, "Session In"=w50) -> ("error out"=w52:errorcluster)  [unwired: 9 in]
  n164 = call "IMAQ Dispose"("error in (no error)"=w52) -> ("error out"=w54:errorcluster)  [unwired: 5 in]
  n165 = Close Python Session(session in=w55, error in=w54) -> (11:w42:errorcluster)
  n166 = shared-variable ".\\Maintenance.lvlib\\error_85"(w42) -> ()  [unwired: 1 in, 1 out]
  "Live Result" <- "Live Result" ("Live Result")
  "Average Result" <- "Average Result" ("Average Result")
  "disc name" <- "Live Info Disc 01" ("Live Result")
  "dsgs" <- "DSGS" ("Live Result")
